vi "SyntaxCheck.vi"(8 "error in":errorcluster, 11 "Parsed Expression In":T1) -> (0 "error out":errorcluster, 1 "Error Index":i32, 2 "Funcion Analizada":string, 3 "Parsed Expression Out":T1)   [LabVIEW 2014, in "MathLoop.lvlib"]
uses:
  MathLoop.lvlib
  TypeDefs/ParsedExpression.ctl
  TypeDefs/typeMed.ctl
  <vilib>/regexp/Match Regular Expression.xnode
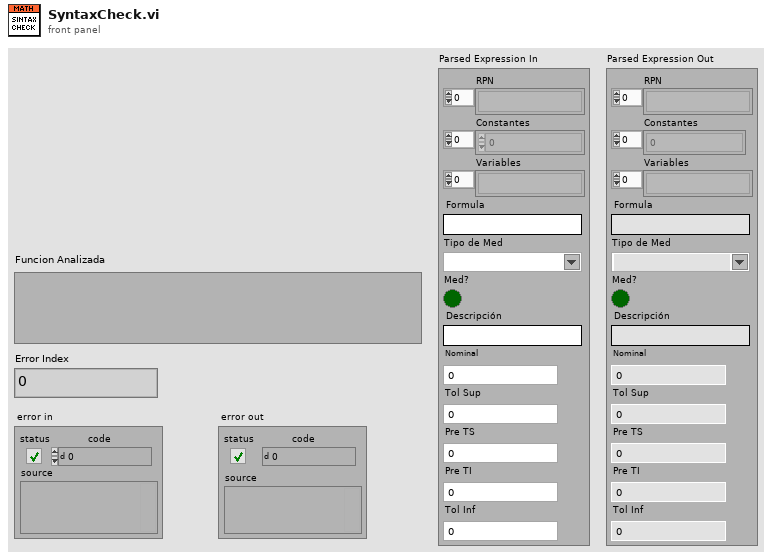
[diagram p1: front panel]
types:
  T1 = typedef "MathLoop.lvlib/ParsedExpression.ctl" = cluster{"RPN ":string[], "Constantes":sgl[], "Variables":string[], "Formula":string, "Tipo de Med":T2, "Med?":bool, "Descripción":string, "Nominal":sgl, "Tol Sup":sgl, "Pre TS":sgl, "Pre TI":sgl, "Tol Inf":sgl}
  T2 = typedef "MathLoop.lvlib/typeMed.ctl" = string
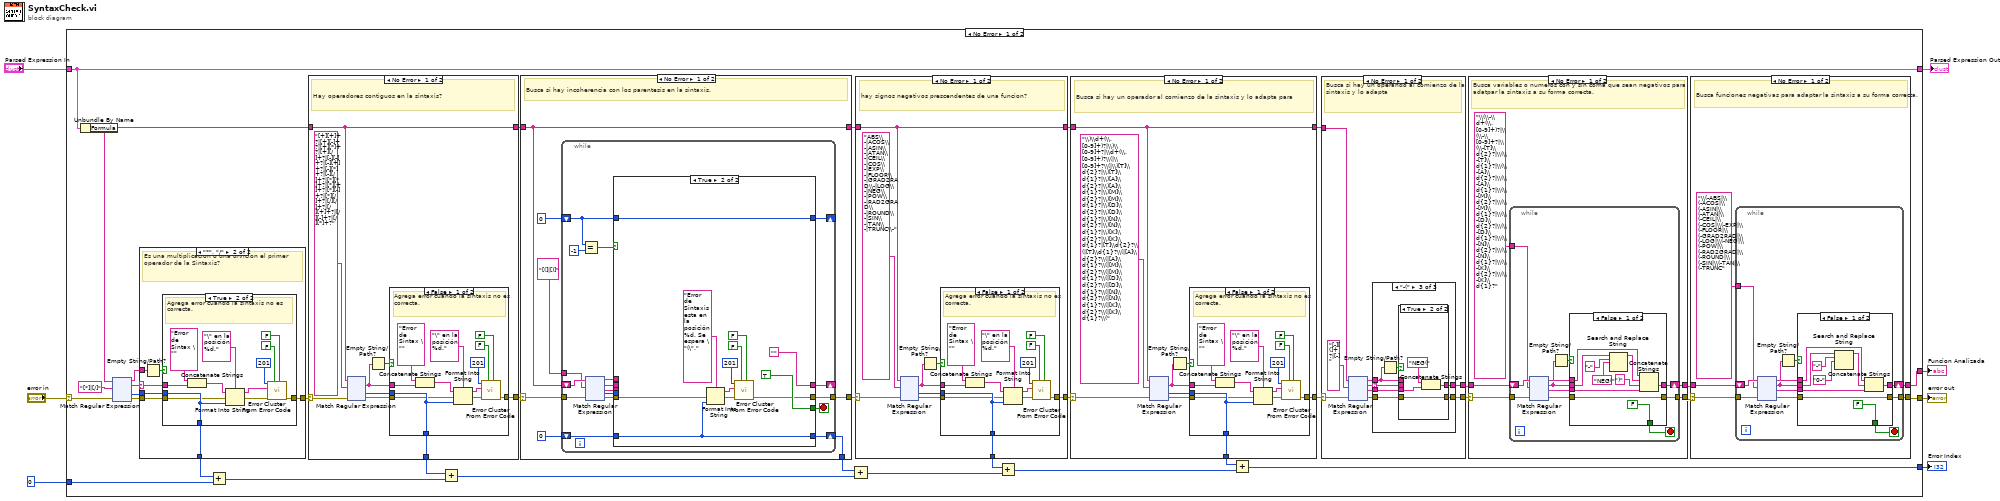
[diagram p0: block diagram]
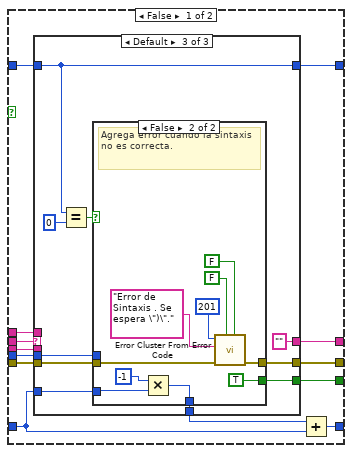
[diagram p2: hidden frame]
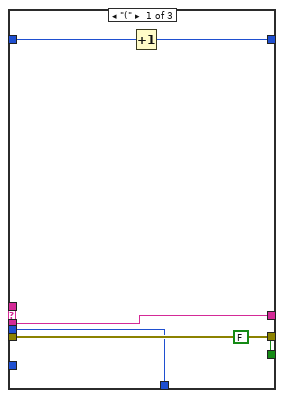
[diagram p3: hidden frame]
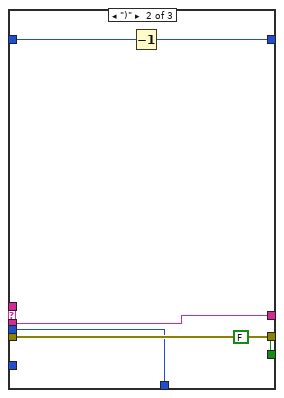
[diagram p4: hidden frame]
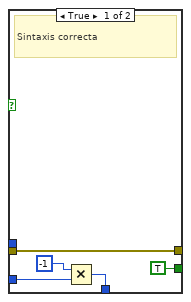
[diagram p5: hidden frame]
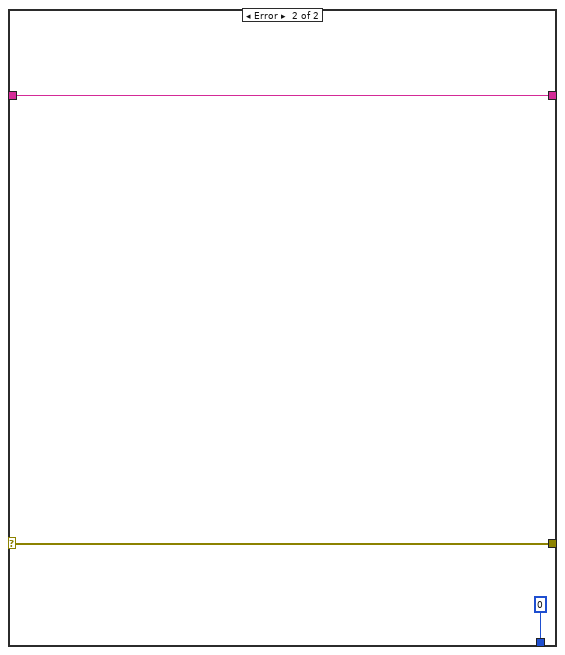
[diagram p6: hidden frame]
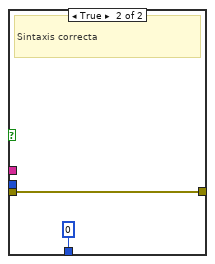
[diagram p7: hidden frame]
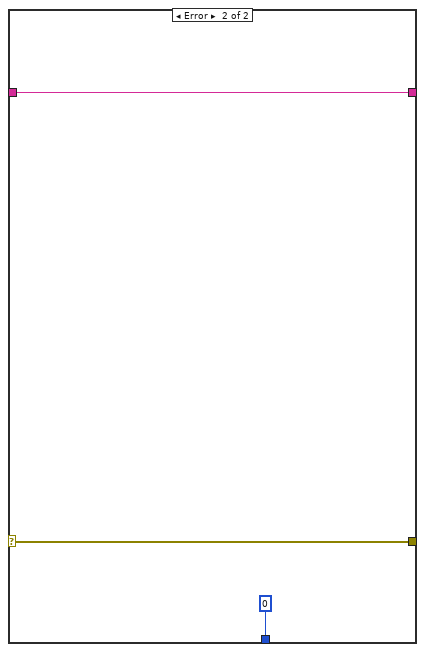
[diagram p8: hidden frame]
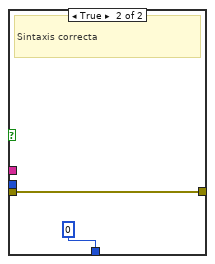
[diagram p9: hidden frame]
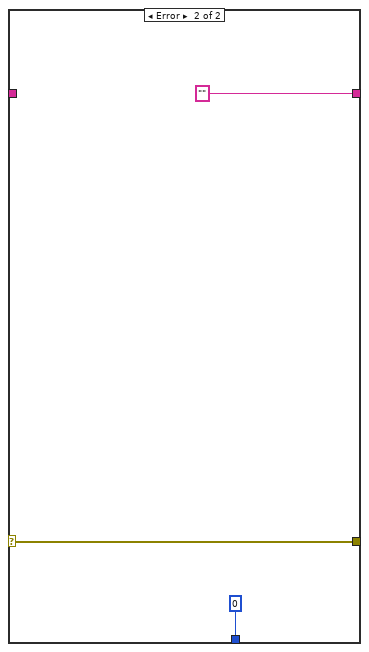
[diagram p10: hidden frame]
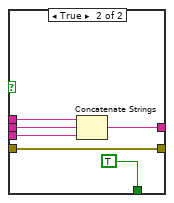
[diagram p11: hidden frame]
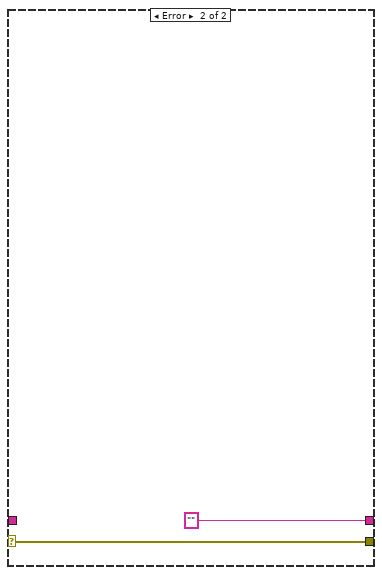
[diagram p12: hidden frame]
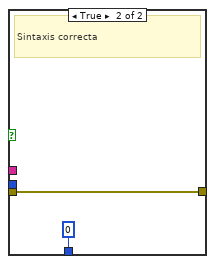
[diagram p13: hidden frame]
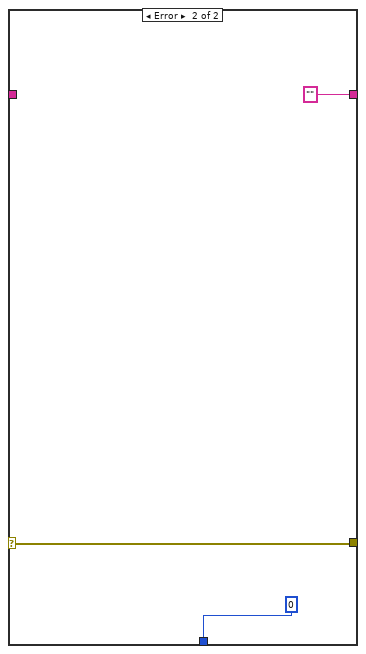
[diagram p14: hidden frame]
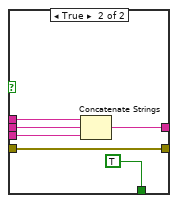
[diagram p15: hidden frame]
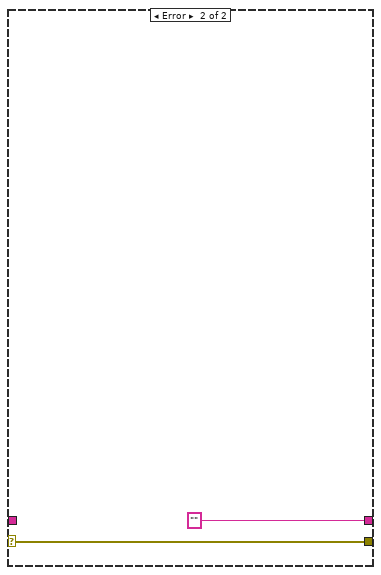
[diagram p16: hidden frame]
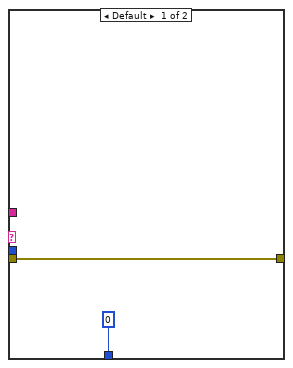
[diagram p17: hidden frame]
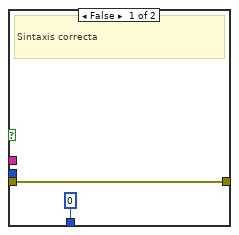
[diagram p18: hidden frame]
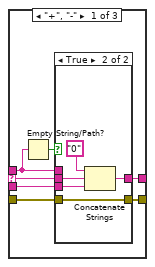
[diagram p19: hidden frame]
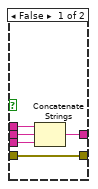
[diagram p20: hidden frame]
diagram:
  n1 = case shown="No Error" "error in" {
    selector: "error in" -> [w37 w1263]
    tunnel: [w33 w1263] -> w7
    tunnel: 0 ("Error Index") -> [w29 _]
    tunnel: "Parsed Expression In" -> [w23 w1262]
    tunnel: [w23 w1262] -> w2
    tunnel: [w24 ""] -> w4
    tunnel: [w16 0] -> w3
    frame No Error {
      n2 = Unbundle By Name(w23) -> ("Formula"=w25:string)
      n3 = xnode "Match Regular Expression"("input string"=w25, "regular expression"="[*]|[/]", "error in"=w37) -> ("before match"=w41:string, "whole match"=w40:string, "offset past match"=w30:i32, "error out"=w39:errorcluster)  [unwired: 3 in, 1 out]
      n4 = case shown="\"*\", \"/\"" w40 {
        selector: w40 -> [_ w966]
        tunnel: w39 -> [w961 w968]
        tunnel: [w961 w967] -> w36
        tunnel: w41 -> [_ w964]
        tunnel: w30 -> [_ w963]
        tunnel: [0 ("offset past match") w962] -> w8
        frame Default {
        }
        frame "*", "/" {
          # "Es una multiplicacion o una divicion el primer operador de la Sintaxis?"
          n5 = Empty String/Path?(string/path=w964) -> (empty?=w965:bool)
          n6 = case shown="True" w965 {
            tunnel: w968 -> [w970 w973]
            tunnel: [w970 w971] -> w967
            tunnel: w966 -> [_ w972]
            tunnel: w963 -> [_ w974]
            tunnel: [0 ("offset past match") w974] -> w962
            frame False {
              # "Sintaxis correcta"
            }
            frame True {
              # "Agrega error cuando la sintaxis no es correcta."
              n7 = Concatenate Strings("Error de Sintax \"" ("error message (\"\")"), w972) -> (w981:string)
              n8 = Format Into String(format string="\" en la posición %d.", initial string=w981, error in=w973, w974) -> (resulting string=w980:string, error out=w979:errorcluster)
              n9 = call <vilib>:"Error Cluster From Error Code.vi"("is warning? (False)"=FALSE, "show call chain? (False)"=FALSE, "error in (no error)"=w979, "error message (\"\")"=w980, "error code (0)"=201) -> ("error out"=w971:errorcluster)  [unwired: 4 in]
            }
          }
        }
      }
      n10 = Add(x=w8, y=w29) -> (x+y=w28:i32)
      n11 = case shown="No Error" w36 {
        selector: w36 -> [w676 w811]
        tunnel: [w674 w811] -> w14
        tunnel: w25 -> [w675 _]
        tunnel: [w675 "" ("String In")] -> w13
        tunnel: [w672 0 ("offset past match")] -> w27
        frame No Error {
          # "Hay operadores contiguos en la sintaxis?"
          n12 = xnode "Match Regular Expression"("input string"=w675, "regular expression"="[+][+]+?|[+][-]+?|[+][*]+?|[+][/]+?|[-][-]+?|[-][+]+?|[-][*]+?|[-][/]+?|[*][*]+?|[*][+]+?|[*][-]+?|[*][/]+?|[/][/]+?|[/][+]+?|[/][-]+?|[/][*]+?", "error in"=w676) -> ("whole match"=w678:string, "offset past match"=w673:i32, "error out"=w679:errorcluster)  [unwired: 3 in, 2 out]
          n13 = Empty String/Path?(string/path=w678) -> (empty?=w677:bool)
          n14 = case shown="False" w677 {
            tunnel: w679 -> [w685 w694]
            tunnel: [w691 w694] -> w674
            tunnel: w678 -> [w688 _]
            tunnel: w673 -> [w686 _]
            tunnel: [w686 0 ("offset past match")] -> w672
            frame False {
              # "Agrega error cuando la sintaxis no es correcta."
              n15 = Concatenate Strings("Error de Sintax \"" ("error message (\"\")"), w688) -> (w682:string)
              n16 = Format Into String(format string="\" en la posición %d.", initial string=w682, error in=w685, w686) -> (resulting string=w683:string, error out=w684:errorcluster)
              n17 = call <vilib>:"Error Cluster From Error Code.vi"("is warning? (False)"=FALSE, "show call chain? (False)"=FALSE, "error in (no error)"=w684, "error message (\"\")"=w683, "error code (0)"=201) -> ("error out"=w691:errorcluster)  [unwired: 4 in]
            }
            frame True {
              # "Sintaxis correcta"
            }
          }
        }
        frame Error {
        }
      }
      n18 = Add(x=w27, y=w28) -> (x+y=w11:i32)
      n19 = case shown="No Error" w14 {
        selector: w14 -> [w47 w244]
        tunnel: [w48 w244] -> w15
        tunnel: w13 -> [w43 w243]
        tunnel: [w43 w243] -> w12
        tunnel: [w42 0] -> w9
        frame No Error {
          # "Busca si hay incoherencia con los parentesis en la sintaxis."
          n20 = while {
            tunnel: "[(]|[)]" ("regular expression") -> [w62]
            shift-right: [w63] -> _
            shift-left: w43 -> [w65]
            tunnel: w47 -> [w64]
            tunnel: [w57] -> w48
            shift-right: [w58] -> _
            shift-left: 0 -> [w52]
            shift-right: [w49] -> w42
            shift-left: 0 -> [w50]
            stop <- w56 stop-if-true
            n21 = Equal?(x=w52, y=-1) -> (x = y?=w53:bool)
            n22 = xnode "Match Regular Expression"("input string"=w65, "regular expression"=w62, "error in"=w64) -> ("before match"=w59:string, "whole match"=w54:string, "after match"=w61:string, "offset past match"=w55:i32, "error out"=w60:errorcluster)  [unwired: 3 in]
            n23 = case shown="True" w53 {
              tunnel: [w78 "" ("after match")] -> w63
              tunnel: w61 -> [w77 _]
              tunnel: w60 -> [w76 w125]
              tunnel: w59 -> [w75 _]
              tunnel: w52 -> [w74 w118]
              tunnel: [w73 w118] -> w58
              tunnel: [w72 w126] -> w57
              tunnel: [w71 TRUE] -> w56
              tunnel: w55 -> [w70 _]
              tunnel: w54 -> [w69 _]
              tunnel: w50 -> [w66 w116]
              tunnel: [w67 w116] -> w49
              frame False {
                n24 = case shown="Default" w69 {
                  tunnel: [w84 w90 "" ("after match")] -> w78
                  tunnel: w75 -> [_ _ _]
                  tunnel: w77 -> [w84 w90 _]
                  tunnel: w76 -> [w83 w89 w100]
                  tunnel: [w83 w89 w99] -> w72
                  tunnel: [FALSE FALSE w97] -> w71
                  tunnel: w74 -> [w82 w88 w95]
                  tunnel: [w81 w87 w95] -> w73
                  tunnel: w70 -> [w79 w85 w96]
                  tunnel: [w79 w85 w94] -> w68
                  tunnel: w66 -> [_ _ w91]
                  frame "(" {
                    n25 = Increment(x=w82) -> (x+1=w81:i32)
                  }
                  frame ")" {
                    n26 = Decrement(x=w88) -> (x-1=w87:i32)
                  }
                  frame Default {
                    n27 = Equal?(x=w95, y=0) -> (x = y?=w93:bool)
                    n28 = case shown="False" w93 {
                      tunnel: w100 -> [w104 w109]
                      tunnel: [w104 w111] -> w99
                      tunnel: [TRUE TRUE] -> w97
                      tunnel: w96 -> [_ _]
                      tunnel: [w102 w107] -> w94
                      tunnel: w91 -> [w101 w108]
                      frame True {
                        # "Sintaxis correcta"
                        n29 = Multiply(x=-1 ("offset past match"), y=w101) -> (x*y=w102:i32)
                      }
                      frame False {
                        # "Agrega error cuando la sintaxis no es correcta."
                        n30 = Multiply(x=-1, y=w108) -> (x*y=w107:i32)
                        n31 = call <vilib>:"Error Cluster From Error Code.vi"("is warning? (False)"=FALSE, "show call chain? (False)"=FALSE, "error in (no error)"=w109, "error message (\"\")"="Error de Sintaxis . Se espera \")\"." ("format string"), "error code (0)"=201) -> ("error out"=w111:errorcluster)  [unwired: 4 in]
                      }
                    }
                  }
                }
                n32 = Add(x=w68, y=w66) -> (x+y=w67:i32)
              }
              frame True {
                n33 = Format Into String(format string="Error de Sintaxis  esta en la posición %d. Se espera \"(\".", error in=w125, w116) -> (resulting string=w120:string, error out=w121:errorcluster)  [unwired: 1 in]
                n34 = call <vilib>:"Error Cluster From Error Code.vi"("is warning? (False)"=FALSE, "show call chain? (False)"=FALSE, "error in (no error)"=w121, "error message (\"\")"=w120, "error code (0)"=201) -> ("error out"=w126:errorcluster)  [unwired: 4 in]
              }
            }
          }
        }
        frame Error {
        }
      }
      n35 = Add(x=w9, y=w11) -> (x+y=w10:i32)
      n36 = case shown="No Error" w15 {
        selector: w15 -> [w393 w524]
        tunnel: [w390 w524] -> w22
        tunnel: w12 -> [w392 _]
        tunnel: [w392 "" ("String In")] -> w21
        tunnel: [w385 0 ("offset past match")] -> w26
        frame No Error {
          # "hay signos negativos prescendentes de una funcion?"
          n37 = xnode "Match Regular Expression"("input string"=w392, "regular expression"="ABS\\-|ACOS\\-|ASIN\\-|ATAN\\-|CEIL\\-|COS\\-|EXP\\-|FLOOR\\-|GRAD2RAD\\-|LOG\\-|NEG\\-|POW\\-|RAD2GRAD\\-|ROUND\\-|SIN\\-|TAN\\-|TRUNC\\-", "error in"=w393) -> ("whole match"=w388:string, "offset past match"=w386:i32, "error out"=w387:errorcluster)  [unwired: 3 in, 2 out]
          n38 = Empty String/Path?(string/path=w388) -> (empty?=w389:bool)
          n39 = case shown="False" w389 {
            tunnel: w387 -> [w398 w407]
            tunnel: [w404 w407] -> w390
            tunnel: w388 -> [w401 _]
            tunnel: w386 -> [w399 _]
            tunnel: [w399 0 ("offset past match")] -> w385
            frame False {
              # "Agrega error cuando la sintaxis no es correcta."
              n40 = Concatenate Strings("Error de Sintax \"" ("error message (\"\")"), w401) -> (w395:string)
              n41 = Format Into String(format string="\" en la posición %d.", initial string=w395, error in=w398, w399) -> (resulting string=w396:string, error out=w397:errorcluster)
              n42 = call <vilib>:"Error Cluster From Error Code.vi"("is warning? (False)"=FALSE, "show call chain? (False)"=FALSE, "error in (no error)"=w397, "error message (\"\")"=w396, "error code (0)"=201) -> ("error out"=w404:errorcluster)  [unwired: 4 in]
            }
            frame True {
              # "Sintaxis correcta"
            }
          }
        }
        frame Error {
        }
      }
      n43 = Add(x=w26, y=w10) -> (x+y=w17:i32)
      n44 = case shown="No Error" w22 {
        selector: w22 -> [w248 w384]
        tunnel: w21 -> [w247 w383]
        tunnel: [w249 w384] -> w20
        tunnel: [w247 w383] -> w19
        tunnel: [w245 0 ("offset past match")] -> w18
        frame No Error {
          # "Busca si hay un operador al comienzo de la sintaxis y lo adapta para"
          n45 = xnode "Match Regular Expression"("input string"=w247, "regular expression"="\\)\\d+(\\.[0-9]+)?|\\)\\[0-9]+?|\\d+(\\.[0-9]+)?\\(|\\[0-9]+?\\(|\\)[T]\\d{2}?|\\)[T]\\d{1}?|\\)[A]\\d{2}?|\\)[A]\\d{1}?|\\)[M]\\d{2}?|\\)[M]\\d{1}?|\\)[D]\\d{2}?|\\)[D]\\d{1}?|\\)[N]\\d{2}?|\\)[N]\\d{1}?|\\)[K]\\d{2}?|\\)[K]\\d{1}?|[T]\\d{2}?\\(|[T]\\d{1}?\\(|[A]\\d{2}?\\(|[A]\\d{1}?\\(|[M]\\d{2}?\\(|[M]\\d{1}?\\(|[D]\\d{2}?\\(|[D]\\d{1}?\\(|[N]\\d{2}?\\(|[N]\\d{1}?\\(|[K]\\d{2}?\\(|[K]\\d{1}?\\(", "error in"=w248) -> ("whole match"=w251:string, "offset past match"=w253:i32, "error out"=w252:errorcluster)  [unwired: 3 in, 2 out]
          n46 = Empty String/Path?(string/path=w251) -> (empty?=w250:bool)
          n47 = case shown="False" w250 {
            tunnel: w252 -> [w258 w267]
            tunnel: [w264 w267] -> w249
            tunnel: w251 -> [w261 _]
            tunnel: w253 -> [w259 _]
            tunnel: [w259 0 ("offset past match")] -> w245
            frame False {
              # "Agrega error cuando la sintaxis no es correcta."
              n48 = Concatenate Strings("Error de Sintax \"" ("error message (\"\")"), w261) -> (w255:string)
              n49 = Format Into String(format string="\" en la posición %d.", initial string=w255, error in=w258, w259) -> (resulting string=w256:string, error out=w257:errorcluster)
              n50 = call <vilib>:"Error Cluster From Error Code.vi"("is warning? (False)"=FALSE, "show call chain? (False)"=FALSE, "error in (no error)"=w257, "error message (\"\")"=w256, "error code (0)"=201) -> ("error out"=w264:errorcluster)  [unwired: 4 in]
            }
            frame True {
              # "Sintaxis correcta"
            }
          }
        }
        frame Error {
        }
      }
      n51 = Add(x=w18, y=w17) -> (x+y=w16:i32)
      n52 = case shown="No Error" w20 {
        selector: w20 -> [w1103 w1259]
        tunnel: w19 -> [w1104 _]
        tunnel: [w1102 w1259] -> w31
        tunnel: [w1101 ""] -> w32
        frame No Error {
          # "Busca si hay un operando al comienzo de la sintaxis y lo adapta"
          n53 = xnode "Match Regular Expression"("input string"=w1104, "regular expression"="[-][(]+?|[-]", "error in"=w1103) -> ("before match"=w1099:string, "whole match"=w1097:string, "after match"=w1100:string, "error out"=w1098:errorcluster)  [unwired: 3 in, 1 out]
          n54 = case shown="\"-(\"" w1097 {
            selector: w1097 -> [w1111 w1123 w1128]
            tunnel: w1100 -> [w1106 w1124 w1133]
            tunnel: w1099 -> [w1107 w1125 w1132]
            tunnel: w1098 -> [w1110 w1127 w1131]
            tunnel: [w1109 w1127 w1130] -> w1102
            tunnel: [w1108 w1126 w1129] -> w1101
            frame "+", "-" {
              n55 = Empty String/Path?(string/path=w1107) -> (empty?=w1112:bool)
              n56 = case shown="True" w1112 {
                tunnel: w1111 -> [w1116 w1118]
                tunnel: w1106 -> [w1115 w1119]
                tunnel: w1107 -> [w1117 _]
                tunnel: [w1114 w1122] -> w1108
                tunnel: [w1113 w1121] -> w1109
                tunnel: w1110 -> [w1113 w1121]
                frame False {
                  n57 = Concatenate Strings(w1117, w1116, w1115) -> (w1114:string)
                }
                frame True {
                  n58 = Concatenate Strings("0" ("string"), w1118, w1119) -> (w1122:string)
                }
              }
            }
            frame Default {
              n59 = Concatenate Strings(w1125, w1123, w1124) -> (w1126:string)
            }
            frame "-(" {
              n60 = Empty String/Path?(string/path=w1132) -> (empty?=w1134:bool)
              n61 = case shown="True" w1134 {
                tunnel: w1128 -> [w1138 _]
                tunnel: w1133 -> [w1137 w1143]
                tunnel: w1132 -> [w1139 _]
                tunnel: [w1136 w1142] -> w1129
                tunnel: [w1135 w1140] -> w1130
                tunnel: w1131 -> [w1135 w1140]
                frame False {
                  n62 = Concatenate Strings(w1139, w1138, w1137) -> (w1136:string)
                }
                frame True {
                  n63 = Concatenate Strings("NEG(" ("string"), w1143) -> (w1142:string)
                }
              }
            }
          }
        }
        frame Error {
        }
      }
      n64 = case shown="No Error" w31 {
        selector: w31 -> [w814 w959]
        tunnel: w32 -> [w816 _]
        tunnel: [w815 w959] -> w35
        tunnel: [w813 ""] -> w34
        frame No Error {
          # "Busca variables o numeros con y sin coma que sean negativos para adatpar la sintaxis a su forma correcta."
          n65 = while {
            tunnel: "\\(\\-\\d+(\\.[0-9]+)?|\\(\\-\\[0-9]+?|\\(\\-[T]\\d{2}?|\\(\\-[T]\\d{1}?|\\(\\-[A]\\d{2}?|\\(\\-[A]\\d{1}?|\\(\\-[M]\\d{2}?|\\(\\-[M]\\d{1}?|\\(\\-[D]\\d{2}?|\\(\\-[D]\\d{1}?|\\(\\-[N]\\d{2}?|\\(\\-[N]\\d{1}?|\\(\\-[K]\\d{2}?|\\(\\-[K]\\d{1}?" ("regular expression") -> [w824]
            shift-right: [w825] -> w813
            shift-left: w816 -> [w827]
            tunnel: w814 -> [w826]
            tunnel: [w820] -> w815
            stop <- w817 stop-if-true
            n66 = xnode "Match Regular Expression"("input string"=w827, "regular expression"=w824, "error in"=w826) -> ("before match"=w823:string, "whole match"=w818:string, "after match"=w822:string, "error out"=w821:errorcluster)  [unwired: 3 in, 1 out]
            n67 = Empty String/Path?(string/path=w818) -> (empty?=w819:bool)
            n68 = case shown="False" w819 {
              tunnel: [w837 w842] -> w825
              tunnel: w818 -> [w836 w840]
              tunnel: w823 -> [w832 w841]
              tunnel: w822 -> [w830 w839]
              tunnel: [w829 w843] -> w820
              tunnel: w821 -> [w829 w843]
              tunnel: [FALSE TRUE] -> w817
              frame False {
                n69 = Search and Replace String(input string=w836, search string="-", replace string="NEG(" ("string")) -> (result string=w833:string)  [unwired: 5 in, 3 out]
                n70 = Concatenate Strings(w832, w833, ")" ("string"), w830) -> (w837:string)
              }
              frame True {
                n71 = Concatenate Strings(w841, w840, w839) -> (w842:string)
              }
            }
          }
        }
        frame Error {
        }
      }
      n72 = case shown="No Error" w35 {
        selector: w35 -> [w527 w671]
        tunnel: w34 -> [w529 _]
        tunnel: [w528 w671] -> w33
        tunnel: [w526 ""] -> w24
        frame No Error {
          # "Busca funciones negativas para adaptar la sintaxis a su forma correcta."
          n73 = while {
            tunnel: "\\(-ABS|\\(-ACOS|\\(-ASIN|\\(-ATAN|\\(-CEIL|\\(-COS|\\(-EXP|\\(-FLOOR|\\(-GRAD2RAD|\\(-LOG|\\(-NEG|\\(-POW|\\(-RAD2GRAD|\\(-ROUND|\\(-SIN|\\(-TAN|\\(-TRUNC" ("regular expression") -> [w537]
            shift-right: [w538] -> w526
            shift-left: w529 -> [w540]
            tunnel: w527 -> [w539]
            tunnel: [w533] -> w528
            stop <- w530 stop-if-true
            n74 = xnode "Match Regular Expression"("input string"=w540, "regular expression"=w537, "error in"=w539) -> ("before match"=w536:string, "whole match"=w531:string, "after match"=w535:string, "error out"=w534:errorcluster)  [unwired: 3 in, 1 out]
            n75 = Empty String/Path?(string/path=w531) -> (empty?=w532:bool)
            n76 = case shown="False" w532 {
              tunnel: [w549 w554] -> w538
              tunnel: w531 -> [w548 w552]
              tunnel: w536 -> [w541 w553]
              tunnel: w535 -> [w545 w551]
              tunnel: [w544 w555] -> w533
              tunnel: w534 -> [w544 w555]
              tunnel: [FALSE TRUE] -> w530
              frame False {
                n77 = Search and Replace String(input string=w548, search string="-", replace string="0-" ("string")) -> (result string=w542:string)  [unwired: 5 in, 3 out]
                n78 = Concatenate Strings(w541, w542, w545) -> (w549:string)
              }
              frame True {
                n79 = Concatenate Strings(w553, w552, w551) -> (w554:string)
              }
            }
          }
        }
        frame Error {
        }
      }
    }
    frame Error {
    }
  }
  "error out" <- w7
  "Funcion Analizada" <- w4
  "Error Index" <- w3
  "Parsed Expression Out" <- w2
